vi "Flock_Shared_WriteDebugMsg.vi"(10 "error in (no error)":errorcluster, 11 "Current Message Case":string) -> (2 "error out":errorcluster)   [LabVIEW 2013, in "Flock_Shared_Messaging.lvlib" / "Flock_Shared_CentralProcessMessaging.lvlib"]
uses:
  Flock_Shared_CentralProcessMessaging.lvlib
  FGV_Action.ctl
  Flock_Shared_Messaging.lvlib
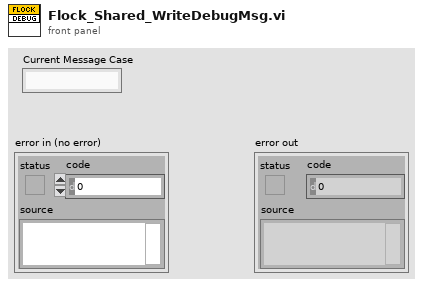
[diagram p1: front panel]
types:
  T1 = typedef "FGV_Action.ctl" = enum16{"Initalize Central", "Initialize Local", "Get", "Delete Local"}
  T2 = typedef "amc_Message Queue.ctl" = refnum<queue>
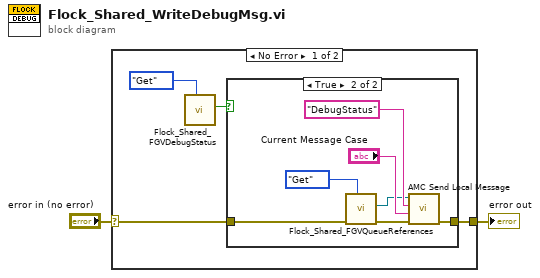
[diagram p0: block diagram]
diagram:
  n1 = case shown="No Error" "error in (no error)" {
    selector: "error in (no error)" -> [w5 w15]
    tunnel: [w6 w15] -> w2
    frame No Error {
      n2 = call "Flock_Shared_FGVDebugStatus.vi"("State"=enum16{"Get", "Set"}."Get") -> ("Debug Boolean"=w3:bool)  [unwired: 10 in]
      n3 = case shown="True" w3 {
        tunnel: [w7 w14] -> w6
        tunnel: w5 -> [w7 w8]
        frame False {
        }
        frame True {
          n4 = call "Flock_Shared_FGVQueueReferences.vi"("Action"=FGV_Action."Get", "error in (no error)"=w8) -> ("error out"=w10:errorcluster, "Central Queue out"=w11:T2)  [unwired: 7 in, 1 out]
          n5 = call <vilib>:"AMC Send Local Message.vi"("error in (no error)"=w10, "Message Value"="Current Message Case", "Message Name"="DebugStatus", "Message Queue in"=w11) -> ("error out"=w14:errorcluster)  [unwired: 6 in, 1 out]
        }
      }
    }
    frame Error {
    }
  }
  "error out" <- w2
